vi "GET.vi"(0 "client handle":T4, 1 "output file":path=path "", 2 "Error code options":T2={"1xx (info)"=FALSE, "2xx (success)"=FALSE, "3xx (redirect)"=FALSE, "4xx (client error)"=TRUE, "5xx (server error)"=TRUE, "Other"=TRUE}, 3 "BlueLogParent in":refnum<class "BlueLogParent_OpenSource.lvclass">, 5 "url":string, 11 "error in (no error)":errorcluster, 12 "timeout (10000)":i32=10000) -> (4 "client handle out":T4, 6 "headers":T3[](array[typedef]), 8 "body":string, 10 "HTTP response code":T1, 15 "error out":errorcluster)   [LabVIEW 2020, in "Blue Easy HTTP OpenSource.lvlib"]
doc: "Sends a Web request that returns headers and body data from a server, Web page, or Web service. This VI uses the GET HTTP method and does not submit any data to the server. You also can save the body data to an output file. Refer to the World Wide Web Consortium Web site at www.w3.org for more information about HTTP method definitions, including the GET method.\n\nYou can assign a client handle to add authentication credentials, HTTP headers, or a cookie to Web requests made by the GET VI. Use the OpenHandle VI to open a client handle and establish credentials. Use the AddHeader VI to add header lines to Web requests made by the GET VI."
uses:
  Blue Easy HTTP OpenSource.lvlib
  <vilib>/httpClient/ClientHandle.ctl
  HTTP Header.ctl
  HTTP error on codes.ctl
  HTTP response code.ctl
  <userlib>/Blue Origin/BlueLogParent_OpenSource/BlueLogParentClass/BlueLogParent_OpenSource.lvclass
  Interpret Header.vi
  <vilib>/dlg_ctls.llb/Space Constant.vi
  <vilib>/Utility/error.llb/Trim Whitespace.vi
  <vilib>/Utility/error.llb/Error Cluster From Error Code.vi
  <vilib>/httpClient/LabVIEWHTTPClient.lvlib
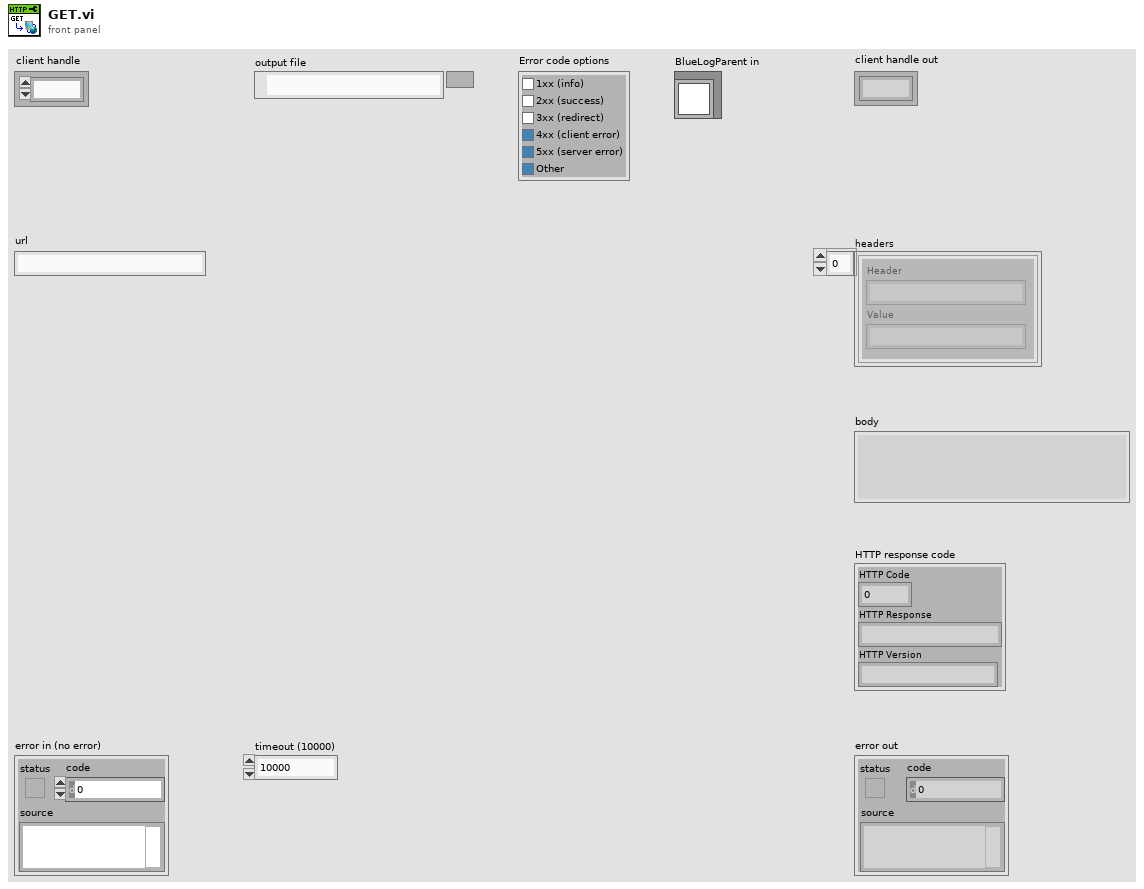
[diagram p1: front panel]
types:
  T1 = typedef "Blue Easy HTTP OpenSource.lvlib/HTTP response code.ctl" = cluster{"HTTP Code":u16, "HTTP Response":string, "HTTP Version":string}
  T2 = typedef "Blue Easy HTTP OpenSource.lvlib/HTTP error on codes.ctl" = cluster{"1xx (info)":bool, "2xx (success)":bool, "3xx (redirect)":bool, "4xx (client error)":bool, "5xx (server error)":bool, "Other":bool}
  T3 = typedef "Blue Easy HTTP OpenSource.lvlib/HTTP Header.ctl" = cluster{"Header":string, "Value":string}
  T4 = typedef "LabVIEWHTTPClient.lvlib/ClientHandle.ctl" = refnum<k1>
  T5 = typedef "BlueLogParent_OpenSource.lvclass/BlueLogParentLevel.ctl" = enum16{"DEBUG", "INFO", "WARNING", "ERROR", "CRITICAL"}
  T6 = typedef "BlueLogParent_OpenSource.lvclass/BlueLogParentOptions.ctl" = cluster{"timestamp (now)":dbl, "Call chain (here)":string, "Count (1)":u16, "Font (override)":T7, "Add row separator? (T)":bool}
  T7 = typedef "BlueLogParent_OpenSource.lvclass/BlueLogParentFont.ctl" = cluster{"Font Name":string, "Size":u16, "Bold":bool, "Italic":bool, "Underline":bool, "Strikeout":bool, "Color":u32}
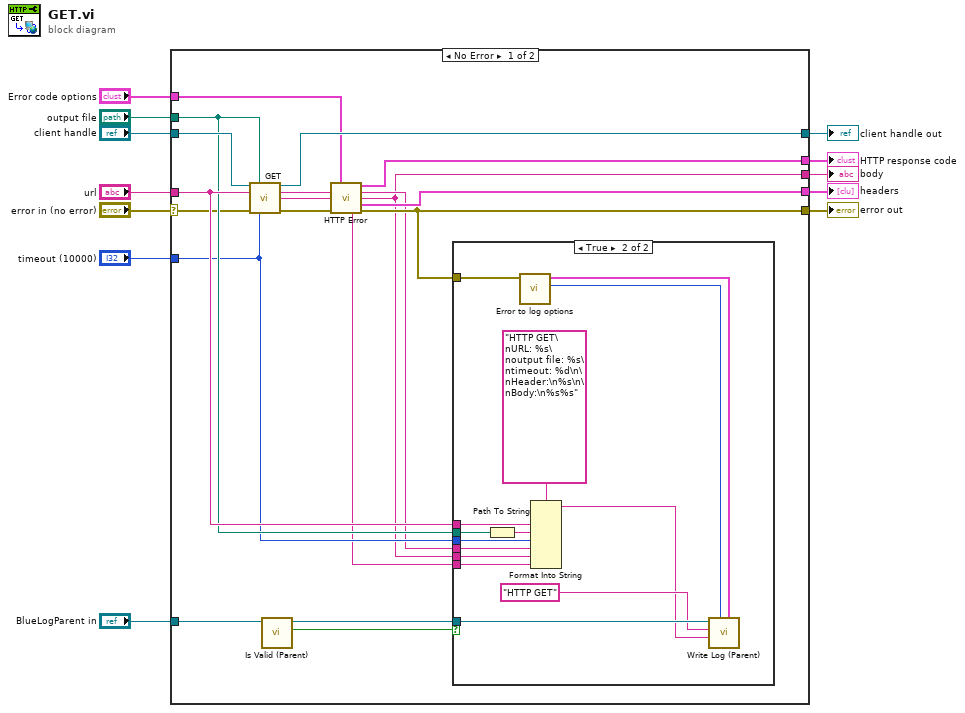
[diagram p0: block diagram]
diagram:
  n1 = case shown="No Error" "error in (no error)" {
    selector: "error in (no error)" -> [w19 w47]
    tunnel: [w28 w47] -> w12
    tunnel: "timeout (10000)" -> [w25 _]
    tunnel: "url" -> [w27 _]
    tunnel: "output file" -> [w26 _]
    tunnel: "client handle" -> [w31 w46]
    tunnel: [w30 w46] -> w6
    tunnel: [w14 _] -> w5
    tunnel: [w23 _] -> w4
    tunnel: "Error code options" -> [w29 _]
    tunnel: [w20 _] -> w2
    tunnel: "BlueLogParent in" -> [w18 _]
    frame No Error {
      n2 = call <vilib>:"GET.vi"("client handle"=w31, "output file"=w26, "url"=w27, "error in (no error)"=w19, "timeout (10000)"=w25) -> ("client handle out"=w30:T4, "headers"=w21:string, "body"=w24:string, "error out"=w22:errorcluster)  [unwired: 7 in]
      n3 = call-dynamic "Is Valid (Parent).vi"("BlueLogParent in"=w18) -> ("Is Valid?"=w17:bool, "BlueLogParent out"=w16:refnum<class "BlueLogParent_OpenSource.lvclass">)  [unwired: 8 in, 1 out]
      n4 = call "HTTP Error.vi"("Error code options"=w29, "Header"=w21, "body"=w24, "error in (no error)"=w22) -> ("HTTP response code"=w20:T1, "Header (dup)"=w15:string, "body (dup)"=w14:string, "Header Values"=w23:T3[], "Error log"=w13:string, "error out"=w28:errorcluster)  [unwired: 6 in]
      n5 = case shown="True" w17 {
        tunnel: w28 -> [_ w37]
        tunnel: w27 -> [_ w44]
        tunnel: w26 -> [_ w43]
        tunnel: w25 -> [_ w41]
        tunnel: w14 -> [_ w40]
        tunnel: w15 -> [_ w39]
        tunnel: w16 -> [_ w38]
        tunnel: w13 -> [_ w32]
        frame False {
        }
        frame True {
          n6 = Path To String(path=w43) -> (string=w42:string)
          n7 = call "Error to log options.vi"("error in (no error)"=w37) -> ("Logging level"=w36:T5, "Options"=w35:T6)  [unwired: 9 in]
          n8 = Format Into String(format string="HTTP GET\nURL: %s\noutput file: %s\ntimeout: %d\n\nHeader:\n%s\n\nBody:\n%s%s", w44, w42, w41, w39, w40, w32) -> (resulting string=w33:string)  [unwired: 2 in, 1 out]
          n9 = call-dynamic "Write Log (Parent).vi"("Options"=w35, "Logging level (INFO)"=w36, "Message"=w33, "Message Title"="HTTP GET" ("Unique ID"), "BlueLogParent in"=w38) -> ()  [unwired: 5 in, 2 out]
        }
      }
    }
    frame Error {
    }
  }
  "error out" <- w12
  "client handle out" <- w6
  "body" <- w5
  "headers" <- w4
  "HTTP response code" <- w2
